vi "Enqueue Message.vi"   [LabVIEW 2023, in "QSM - Limits.lvlib"]
doc: "This polymorphic VI enqueues a message or an array of messages in the message queue for the Queued State Machine template."
uses:
  QSM - Limits.lvlib
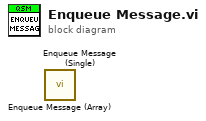
[diagram p0: block diagram]
diagram:
  n1 = call "Enqueue Message (Array).vi"() -> ()  [unwired: 11 in, 1 out]
  n2 = call "Enqueue Message (Single).vi"() -> ()  [unwired: 11 in, 1 out]
